vi "Steinhart.vi"(6 "c":dbl, 7 "R1":dbl, 8 "b":dbl, 9 "a":dbl, 10 "Vex":dbl, 11 "Vm":dbl) -> (2 "output variable":dbl)   [LabVIEW 2017]
panel:
  out "Rm":dbl
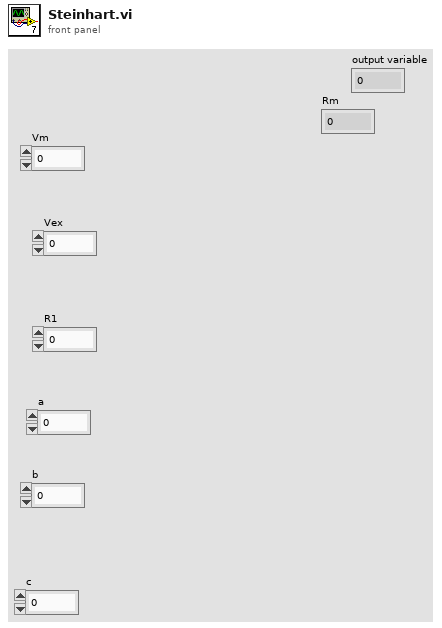
[diagram p1: front panel]
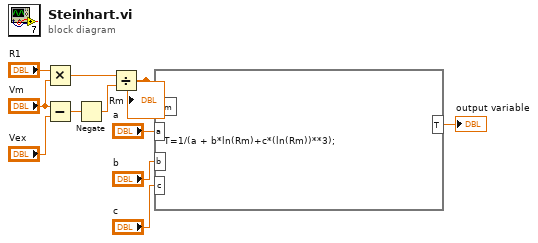
[diagram p0: block diagram]
diagram:
  n1 = Multiply(x="R1", y="Vm") -> (x*y=w7:dbl)
  n2 = Subtract(x="Vm", y="Vex") -> (x-y=w8:dbl)
  n3 = Negate(x=w8) -> (-x=w6:dbl)
  n4 = Divide(x=w7, y=w6) -> (x/y=w5:dbl)
  "Rm" <- w5
  n5 = formula code="T=1/(a + b*ln(Rm)+c*(ln(Rm))**3);"("Rm"=w5, "a"="a", "b"="b", "c"="c") -> ("T"=→"output variable":dbl)
